vi "E4440A_PSA_Configure_Level.vi"(0 "VISA resource name":refnum<visa-resource-name>, 1 "Reference Level (0)":dbl, 2 "Reference Level Offset (0 dB)":dbl, 5 "Amplitude Units (0: dBm)":u16(ring) items=["dBm", "dBmV", "dBmA", "dBuV", "dBuVm", "dBuA", "dBuAm", "dBpt", "dBg", "Volts", "Watts", "Amps"], 11 "error in (no error)":errorcluster, 12 "Enable Auto Attenuation (T: Enable)":bool=TRUE, 13 "Manual Attenuation (30 dB)":dbl=30.0, 14 "Attenuation Step (2 dB)":i32=2) -> (4 "VISA resource name out":refnum<visa-resource-name>, 15 "error out":errorcluster)   [LabVIEW 2015]
doc: "Configures the vertical settings of the spectrum analyzer."
panel:
  # "For PSA"
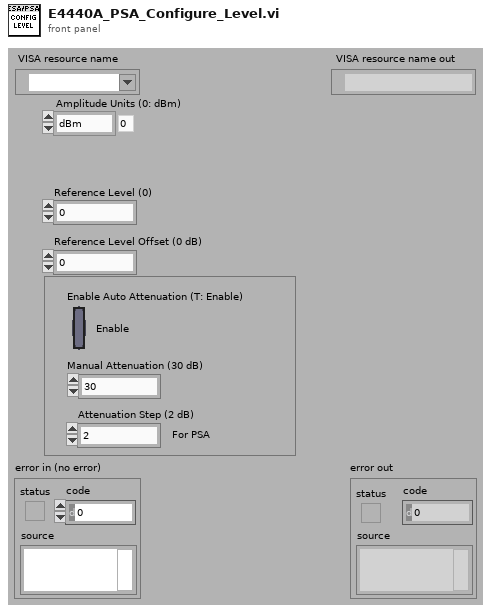
[diagram p1: front panel]
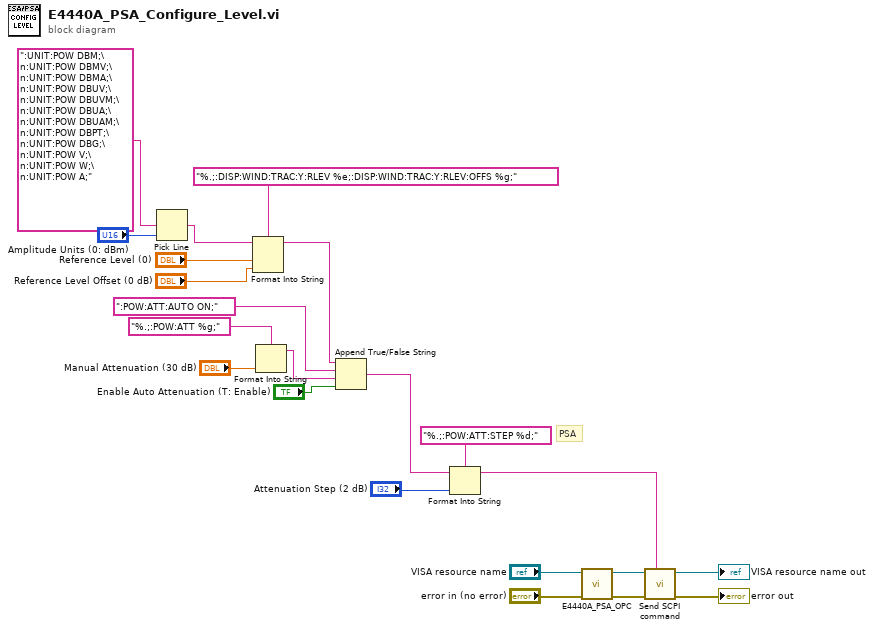
[diagram p0: block diagram]
diagram:
  # "PSA"
  n1 = Pick Line(multi-line string=":UNIT:POW DBM;\n:UNIT:POW DBMV;\n:UNIT:POW DBMA;\n:UNIT:POW DBUV;\n:UNIT:POW DBUVM;\n:UNIT:POW DBUA;\n:UNIT:POW DBUAM;\n:UNIT:POW DBPT;\n:UNIT:POW DBG;\n:UNIT:POW V;\n:UNIT:POW W;\n:UNIT:POW A;", line index="Amplitude Units (0: dBm)") -> (output string=w18:string)  [unwired: 1 in]
  n2 = Format Into String(format string="%.;:DISP:WIND:TRAC:Y:RLEV %e;:DISP:WIND:TRAC:Y:RLEV:OFFS %g;", initial string=w18, "Reference Level (0)", "Reference Level Offset (0 dB)") -> (resulting string=w11:string)  [unwired: 1 in, 1 out]
  n3 = Format Into String(format string="%.;:POW:ATT %g;", "Manual Attenuation (30 dB)") -> (resulting string=w13:string)  [unwired: 2 in, 1 out]
  n4 = Append True/False String(1:"Enable Auto Attenuation (T: Enable)", 2:w13, 3:":POW:ATT:AUTO ON;" ("string (\"\")"), 4:w11) -> (0:w9:string)
  n5 = Format Into String(format string="%.;:POW:ATT:STEP %d;", initial string=w9, "Attenuation Step (2 dB)") -> (resulting string=w4:string)  [unwired: 1 in, 1 out]
  n6 = call "E4440A_PSA_OPC.vi"("error in (no error)"="error in (no error)", "VISA resource name"="VISA resource name") -> ("error out"=w3:errorcluster, "VISA resource name out"=w1:refnum<visa-resource-name>)  [unwired: 8 in]
  n7 = call "Send SCPI command.vi"("Send SCPI Command"=w4, "error in (no error)"=w3, "VISA resource name"=w1) -> ("error out"=→"error out":errorcluster, "VISA resource name out"=→"VISA resource name out":refnum<visa-resource-name>)  [unwired: 7 in]
